vi "TEST Text to Timestamp.vi"() -> ()   [LabVIEW 2020]
uses:
  <vilib>/JDP Science/JDP Science Common Utilities/Timestamp/JDP Timestamp.lvlib
panel:
  out "Timestamps 2":timestamp[](array[timestamp]) format="%^<%.9X %x>T"
  out "Should be ERROR":errorcluster[](array[cluster])
  out "OK":bool[](array[boolean])
  out "Should be NO Error":errorcluster[](array[cluster])
  out "Timestamps":timestamp[](array[timestamp]) format="%^<%.9X %x>T"
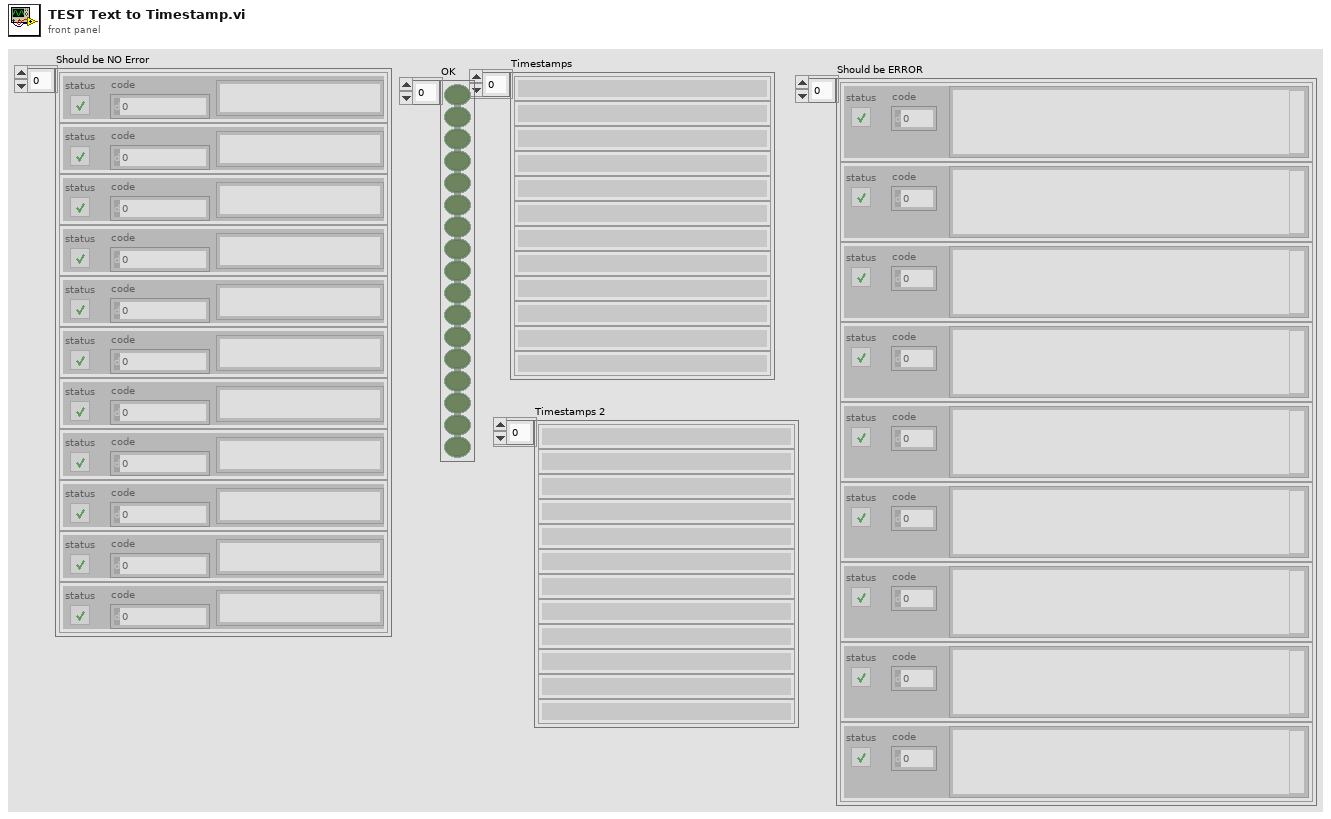
[diagram p1: front panel]
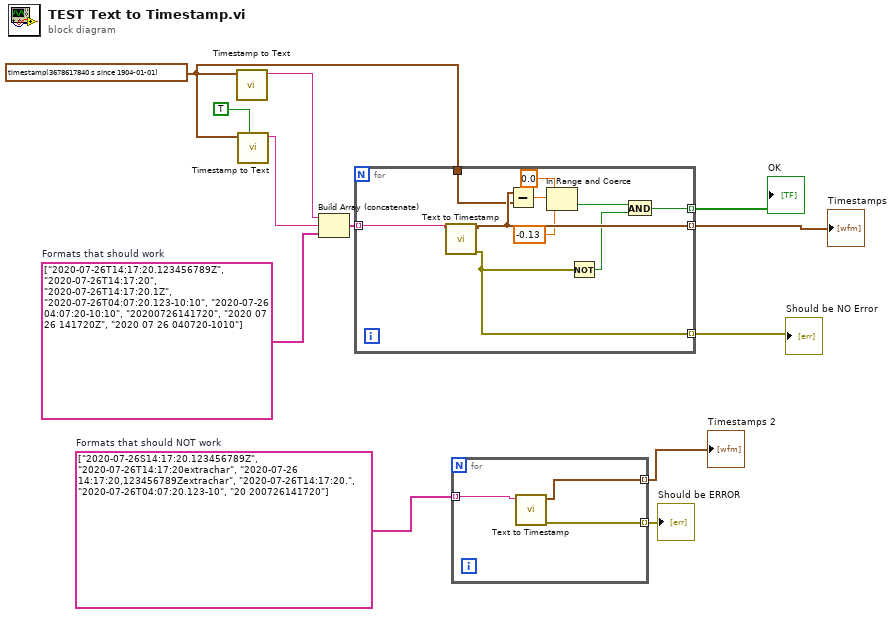
[diagram p0: block diagram]
diagram:
  w3 = string[] ["2020-07-26S14:17:20.123456789Z", "2020-07-26T14:17:20extrachar", "2020-07-26 14:17:20,123456789Zextrachar", "2020-07-26T14:17:20.", "2020-07-26T04:07:20.123-10", "20 200726141720"]  # Formats that should NOT work
  w5 = timestamp(3678617840.123457 s since 1904-01-01) ("Time Stamp")
  w12 = string[] ["2020-07-26T14:17:20.123456789Z", "2020-07-26T14:17:20", "2020-07-26T14:17:20.1Z", "2020-07-26T04:07:20.123-10:10", "2020-07-26 04:07:20-10:10", "20200726141720", "2020 07 26 141720Z", "2020 07 26 040720-1010"]  # Formats that should work
  n1 = call <vilib>:"Timestamp to Text.vi"("Time Stamp"=w5) -> ("Timestamp (RFC3339)"=w8:string)  [unwired: 9 in, 1 out]
  n2 = call <vilib>:"Timestamp to Text.vi"("Local Time Offset format"=TRUE, "Time Stamp"=w5) -> ("Timestamp (RFC3339)"=w6:string)  [unwired: 8 in, 1 out]
  n3 = Build Array (concatenate)(w8, w6, w12) -> (w9:string[])
  n4 = for {
    tunnel: w9 -> [w22] mode=indexing
    tunnel: [w21] -> w11 mode=indexing
    tunnel: [w15] -> w10 mode=indexing
    tunnel: w5 -> [w20]
    tunnel: [w13] -> w4 mode=indexing
    n5 = call <vilib>:"Text to Timestamp.vi"("Text Timestamp"=w22) -> ("error out"=w15:errorcluster, "Time Stamp"=w21:timestamp)  [unwired: 7 in, 2 out]
    n6 = Subtract(x=w21, y=w20) -> (x-y=w19:dbl)
    n7 = In Range and Coerce(upper limit=0.0, x=w19, lower limit=-0.13) -> (In Range?=w16:bool)  [unwired: 1 out]
    n8 = Not(x=w15) -> (.not. x?=w14:bool)
    n9 = And(x=w16, y=w14) -> (x .and. y?=w13:bool)
  }
  "Timestamps" <- w11
  "Should be NO Error" <- w10
  "OK" <- w4
  n10 = for {
    tunnel: w3 -> [w25] mode=indexing
    tunnel: [w24] -> w2 mode=indexing
    tunnel: [w23] -> w1 mode=indexing
    n11 = call <vilib>:"Text to Timestamp.vi"("Text Timestamp"=w25) -> ("error out"=w24:errorcluster, "Time Stamp"=w23:timestamp)  [unwired: 7 in, 2 out]
  }
  "Should be ERROR" <- w2
  "Timestamps 2" <- w1
